vi "Particle Classifier.vi"(4 "camResY":dbl, 5 "vert":dbl, 6 "camResX":dbl, 7 "horz":dbl, 8 "BndRectBtm":dbl, 9 "BndRectRight":dbl, 10 "BndRectLeft":dbl, 11 "BndRectTop":dbl) -> (2 "class":i32)   [LabVIEW 2012]
panel:
  # "INPUTS"
  # "OUTPUTS"
  # "Average Segment Length"
  # "Classification System\n0- Undefined/Drivers Station Stripe (default)\n1- One Point Goal\n2- Two Point Goal (Left or Right)\n3- Three Point Goal\n4- Touching Edge i.e. AR Invalid"
  # "Camera Resolution"
  # "Bounding Rectangle"
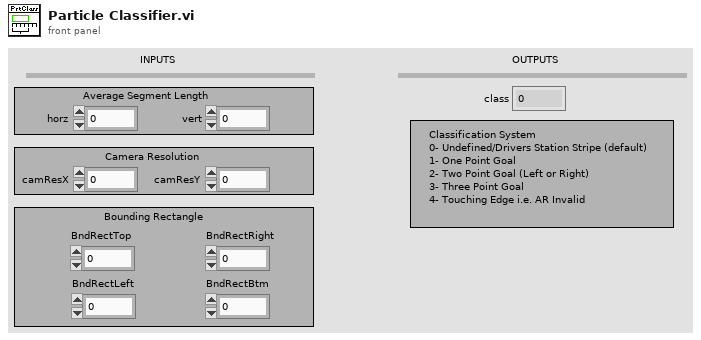
[diagram p1: front panel]
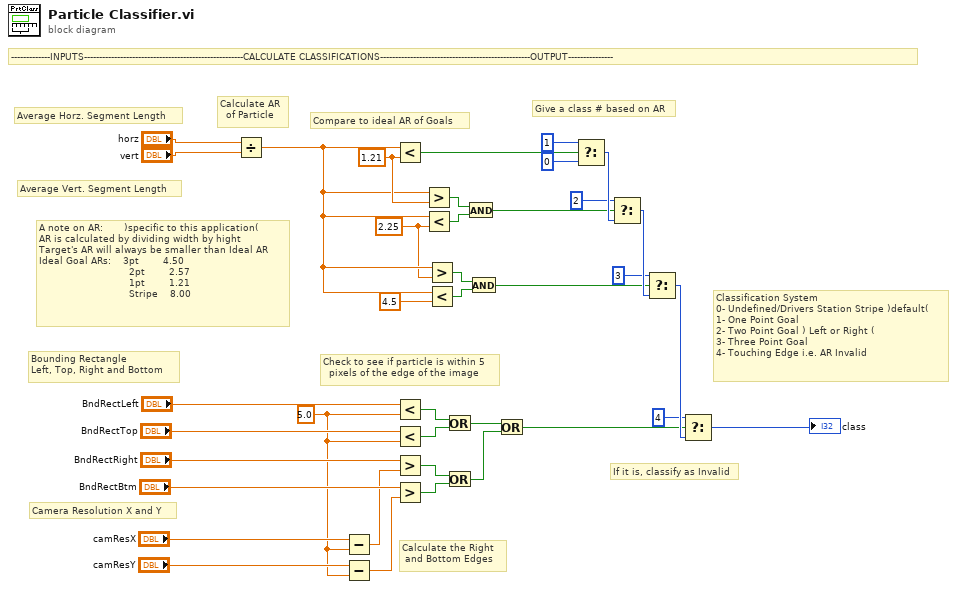
[diagram p0: block diagram]
diagram:
  w6 = 5.0 ("y")
  w22 = 2.25 ("y")
  w30 = 1.21 ("y")
  # "-------------INPUTS-----------------------------------------------------CALCULATE CLASSIFICATIONS--------------------------------------------------OUTPUT---------------"
  # "Calculate the Right \n and Bottom Edges"
  # "Camera Resolution X and Y"
  # "A note on AR:       )specific to this application(\nAR is calculated by dividing width by hight\nTarget's AR will always be smaller than Ideal AR\nIdeal Goal ARs:    3pt        4.50\n                              2pt        2.57\n                              1pt        1.21\n                              Stripe    8.00"
  # "If it is, classify as Invalid"
  # "Check to see if particle is within 5\n  pixels of the edge of the image"
  # "Bounding Rectangle\nLeft, Top, Right and Bottom"
  # "Average Vert. Segment Length"
  # "Average Horz. Segment Length"
  # "Give a class # based on AR"
  # "Compare to ideal AR of Goals"
  # "Calculate AR\n  of Particle"
  # "Classification System\n0- Undefined/Drivers Station Stripe )default(\n1- One Point Goal\n2- Two Point Goal ) Left or Right (\n3- Three Point Goal\n4- Touching Edge i.e. AR Invalid"
  n1 = Divide(x="horz", y="vert") -> (x/y=w23:dbl)
  n2 = Subtract(x="camResX", y=w6) -> (x-y=w5:dbl)
  n3 = Subtract(x="camResY", y=w6) -> (x-y=w4:dbl)
  n4 = Less?(x=w23, y=w30) -> (x < y?=w33:bool)
  n5 = Less?(x="BndRectLeft", y=w6) -> (x < y?=w17:bool)
  n6 = Less?(x="BndRectTop", y=w6) -> (x < y?=w18:bool)
  n7 = Greater?(x="BndRectRight", y=w5) -> (0:w13:bool)
  n8 = Greater?(x="BndRectBtm", y=w4) -> (0:w14:bool)
  n9 = Greater?(x=w23, y=w30) -> (0:w29:bool)
  n10 = Less?(x=w23, y=w22) -> (x < y?=w28:bool)
  n11 = Greater?(x=w23, y=w22) -> (0:w26:bool)
  n12 = Less?(x=w23, y=4.5) -> (x < y?=w25:bool)
  n13 = Or(x=w17, y=w18) -> (x .or. y?=w11:bool)
  n14 = Or(x=w13, y=w14) -> (x .or. y?=w10:bool)
  n15 = And(x=w29, y=w28) -> (x .and. y?=w27:bool)
  n16 = And(x=w26, y=w25) -> (x .and. y?=w24:bool)
  n17 = Or(x=w11, y=w10) -> (x .or. y?=w12:bool)
  n18 = Select(t=1, s=w33, f=0) -> (s? t:f=w38:i32)
  n19 = Select(t=2 ("f"), s=w27, f=w38) -> (s? t:f=w37:i32)
  n20 = Select(t=3 ("f"), s=w24, f=w37) -> (s? t:f=w36:i32)
  n21 = Select(t=4 ("f"), s=w12, f=w36) -> (s? t:f=→"class":i32)
